vi "Var to Boolean.vi"(11 "Variant":variant) -> (3 "Boolean":bool)   [LabVIEW 2019]
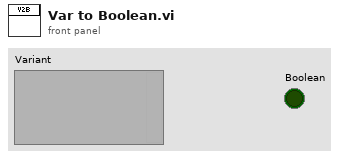
[diagram p1: front panel]
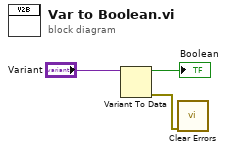
[diagram p0: block diagram]
diagram:
  n1 = Variant To Data(Variant="Variant") -> (data=→"Boolean":bool, error out=w2:errorcluster)  [unwired: 2 in]
  n2 = call <vilib>:"Clear Errors.vi"("error in (no error)"=w2) -> ()  [unwired: 5 in, 2 out]
